vi "log error.vi"(8 "error in":errorcluster, 11 "message":string) -> (0 "error out":errorcluster)   [LabVIEW 2019]
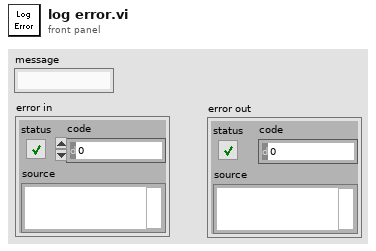
[diagram p1: front panel]
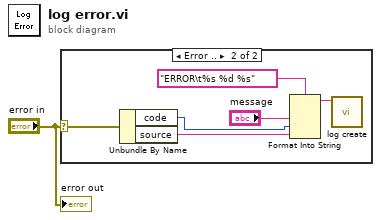
[diagram p0: block diagram]
diagram:
  n1 = case shown="Error .." "error in" {
    selector: "error in" -> [_ w7]
    frame No Error {
    }
    frame Error {
      n2 = Unbundle By Name(w7) -> ("code"=w4:i32, "source"=w5:string)
      n3 = Format Into String(format string="ERROR\t%s %d %s", "message", w4, w5) -> (resulting string=w2:string)  [unwired: 2 in, 1 out]
      n4 = call "log create.vi"("message"=w2) -> ()  [unwired: 11 in]
    }
  }
  "error out" <- "error in"
